vi "Read Trace Buffer Statistic.vi"(8 "error in (no error)":errorcluster, 9 "Statistical Operation (2: MEAN)":i32(ring)=2 items=["SDEV", "PKPK", "MEAN", "MIN", "MAX"], 10 "Channel (0: Channel 1)":i32(ring) items=["Channel 1", "Channel 2"], 11 "VISA resource name":refnum<visa-resource-name>) -> (0 "error out":errorcluster, 2 "Trace Buffer Data Statistical Result":dbl, 3 "VISA resource name out":refnum<visa-resource-name>)   [LabVIEW 2020, in "Agilent B2900 Series.lvlib"]
doc: "Reads the result of the statistical operation for the data stored in the trace buffer."
uses:
  Agilent B2900 Series.lvlib
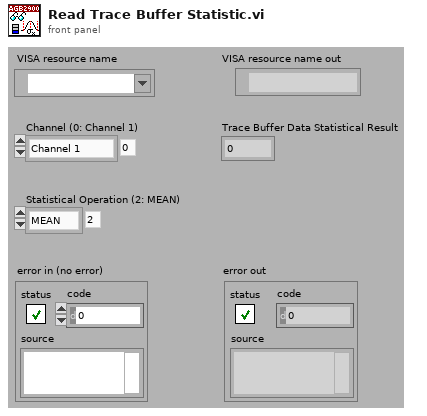
[diagram p1: front panel]
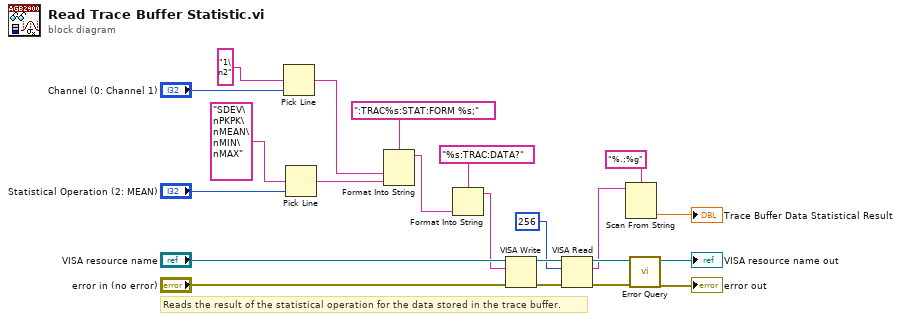
[diagram p0: block diagram]
diagram:
  # "Reads the result of the statistical operation for the data stored in the trace buffer."
  n1 = Pick Line(multi-line string="1\n2" ("string (\"\")"), line index="Channel (0: Channel 1)") -> (output string=w6:string)  [unwired: 1 in]
  n2 = Pick Line(multi-line string="SDEV\nPKPK\nMEAN\nMIN\nMAX", line index="Statistical Operation (2: MEAN)") -> (output string=w7:string)  [unwired: 1 in]
  n3 = Format Into String(format string=":TRAC%s:STAT:FORM %s;", w6, w7) -> (resulting string=w1:string)  [unwired: 2 in, 1 out]
  n4 = Format Into String(format string="%s:TRAC:DATA?", w1) -> (resulting string=w15:string)  [unwired: 2 in, 1 out]
  n5 = VISA Write(VISA resource name="VISA resource name", write buffer=w15, error in (no error)="error in (no error)") -> (VISA resource name out=w13:refnum<visa-resource-name>, error out=w14:errorcluster)  [unwired: 1 out]
  n6 = VISA Read(VISA resource name=w13, byte count=u32 256, error in (no error)=w14) -> (VISA resource name out=w12:refnum<visa-resource-name>, read buffer=w3:string, error out=w11:errorcluster)  [unwired: 1 out]
  n7 = Scan From String(format string="%.;%g", input string=w3) -> (output 1=→"Trace Buffer Data Statistical Result":dbl)  [unwired: 3 in, 3 out]
  n8 = call "Error Query.vi"("error in (no error)"=w11, "VISA resource name"=w12) -> ("error out"=→"error out":errorcluster, "VISA resource name out"=→"VISA resource name out":refnum<visa-resource-name>)  [unwired: 6 in, 2 out]
